vi "Close.vi"(6 "deadline":T1={"mode"=enum."Relative", "deadline (ms)"=30000}, 8 "error in (no error)":errorcluster, 11 "subprocess in":refnum<class "Subprocess.lvclass">) -> (0 "error out":errorcluster, 2 "return code":u8, 3 "subprocess out":refnum<class "Subprocess.lvclass">)   [LabVIEW 2020, in "NI_Subprocess.lvlib" / "Subprocess.lvclass"]
doc: "Wait for <b>subprocess</b> to terminate, then free its resources."
uses:
  <vilib>/Subprocess/Subprocess/Subprocess.lvclass
  <vilib>/Utility/Deadline/Deadline.ctl
  <vilib>/Utility/Deadline/Mode.ctl
  <vilib>/Subprocess/Subprocess/Subprocess.lvclass/Subprocess.ctl
  <vilib>/Utility/Deadline/NI_Deadline.lvlib
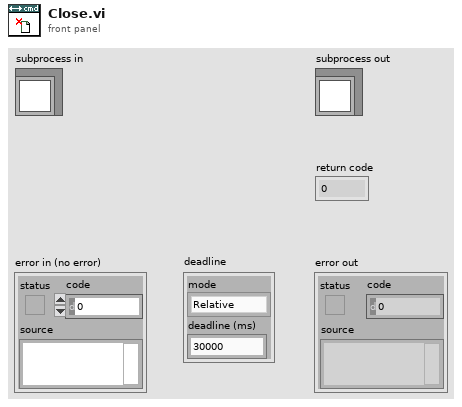
[diagram p1: front panel]
types:
  T1 = typedef "NI_Deadline.lvlib/Deadline.ctl" = cluster{"mode":T2, "deadline (ms)":u32}
  T2 = typedef "NI_Deadline.lvlib/Mode.ctl" = enum16{"Relative", "Use deadline", "Wait forever", "Nonblocking", "N/A"}
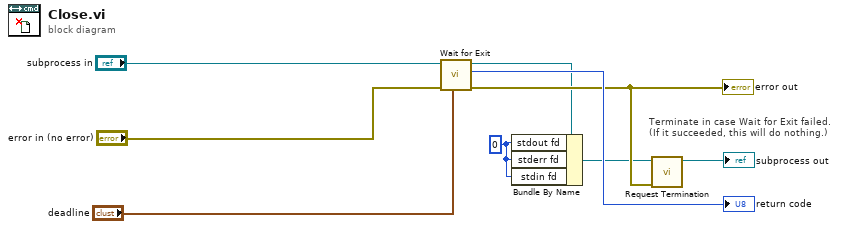
[diagram p0: block diagram]
diagram:
  w9 = u64 0 ("stdout fd")
  # "Terminate in case Wait for Exit failed.\n(If it succeeded, this will do nothing.)"
  n1 = call <vilib>:"Wait for Exit.vi"("deadline"="deadline", "error in (no error)"="error in (no error)", "subprocess in"="subprocess in") -> ("error out"=w5:errorcluster, "return code"=→"return code":u8, "subprocess out"=w4:refnum<class "Subprocess.lvclass">)  [unwired: 6 in]
  "error out" <- w5
  n2 = Bundle By Name(cluster=w4, "stdout fd"=w9, "stderr fd"=w9, "stdin fd"=w9) -> (w3:refnum<class "Subprocess.lvclass">)
  n3 = call <vilib>:"Request Termination.vi"("error in (no error)"=w5, "subprocess in"=w3) -> ("subprocess out"=→"subprocess out":refnum<class "Subprocess.lvclass">)  [unwired: 8 in, 1 out]
